vi "Formal Check Columns by Int.vi"(10 "Sudoku Formal In":T1, 11 "Sudoku Int":u8[][](array[numeric])) -> (2 "Sudoku Formal Out":T1, 3 "Is Modify":bool)   [LabVIEW 2015, in "Sudoku Library.lvlib"]
doc: "Created IvanLis by LabVIEW Portal\nProfile: http://labviewportal.org/memberlist.php?mode=viewprofile&u=987\neMail: IvanLisanov@gMail.com\nTelegram: https://t.me/IvanLis"
uses:
  Sudoku Library.lvlib
  TypeDef/Sudoku Formal.ctl
  TypeDef/Cell Formal.ctl
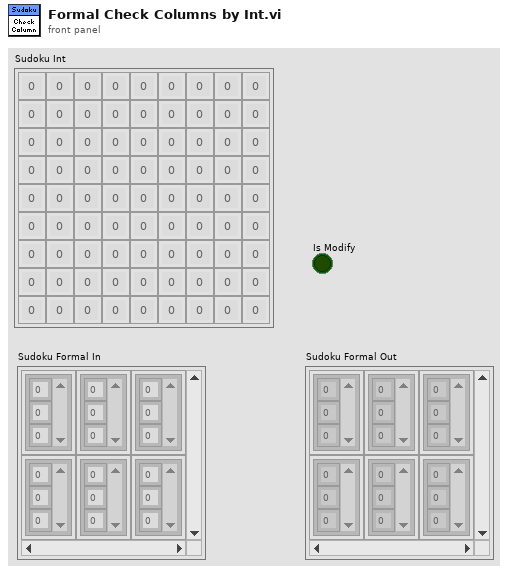
[diagram p1: front panel]
types:
  T1 = typedef "Sudoku Library.lvlib/Sudoku Formal.ctl" = T2[][]
  T2 = typedef "Sudoku Library.lvlib/Cell Formal.ctl" = cluster{"Variant":u8[]}
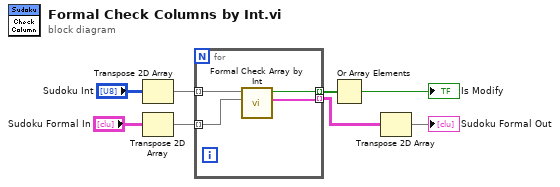
[diagram p0: block diagram]
diagram:
  n1 = Transpose 2D Array(2D array="Sudoku Int") -> (transposed array=w7:u8[][])
  n2 = Transpose 2D Array(2D array="Sudoku Formal In") -> (transposed array=w5:T1)
  n3 = for {
    tunnel: w7 -> [w12] mode=indexing
    tunnel: w5 -> [w11] mode=indexing
    tunnel: [w10] -> w3 mode=indexing
    tunnel: [w9] -> w4 mode=indexing
    n4 = call "Formal Check Array by Int.vi"("Array Formal In"=w11, "Array In"=w12) -> ("Array Formal Out"=w9:T2[], "Is Modify"=w10:bool)  [unwired: 8 in]
  }
  n5 = Or Array Elements(Boolean array=w3) -> (logical OR=→"Is Modify":bool)
  n6 = Transpose 2D Array(2D array=w4) -> (transposed array=→"Sudoku Formal Out":T2[][])
